vi "OpenLogFiles.vi"(8 "error in (no error)":errorcluster, 11 "WORef":T1) -> (0 "error out":errorcluster, 1 "FailRef":refnum<file>, 2 "PassRef":refnum<file>, 3 "WORef Out":T1)   [LabVIEW 2011]
uses:
  Classes/WorkorderHandler/Software/DataStructures/WorkorderHandler_ObjectReference.ctl
  Strict Type Controls/Settings Operation.ctl
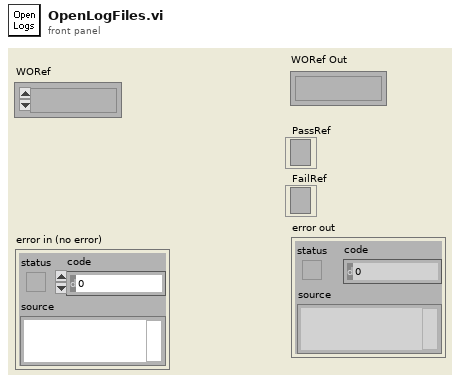
[diagram p1: front panel]
types:
  T1 = typedef "WorkorderHandler_ObjectReference.ctl" = refnum<k1>
  T2 = enum16{"open", "replace", "create", "open or create", "replace or create", "replace or create with confirmation"}
  T3 = typedef "Settings Operation.ctl" = enum8{"Get Value", "Set Value", "Read File", "Write File", "Write Stored Value"}
  T4 = cluster{"PassLog":path, "Fail Log":path, "Header":string, "LastSr":string}
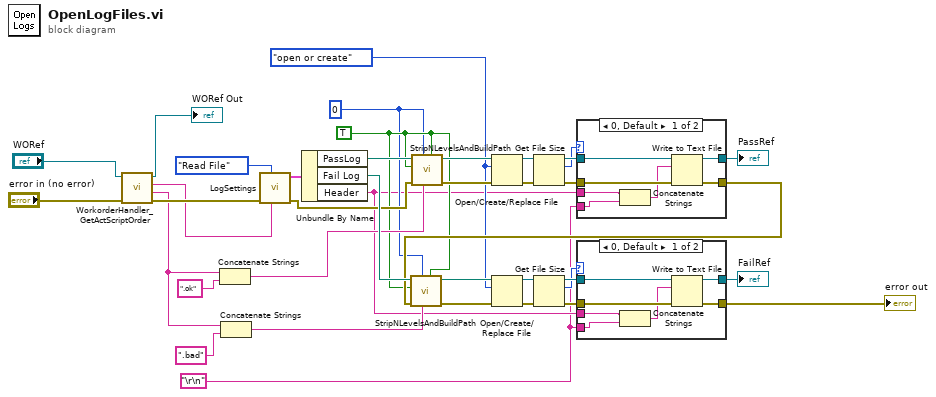
[diagram p0: block diagram]
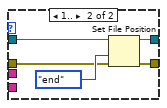
[diagram p2: hidden frame]
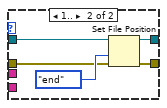
[diagram p3: hidden frame]
diagram:
  w9 = "\r\n"
  w14 = 0 ("Strip Levels")
  w15 = T2."open or create" ("operation (0:open)")
  w17 = TRUE ("Create Folders")
  n1 = call "WorkorderHandler_GetActScriptOrder.vi"("error in (no error)"="error in (no error)", "reference"="WORef") -> ("error out"=w4:errorcluster, "Order"=w2:string, "Script"=w3:string, "duplicate reference"=→"WORef Out":T1)  [unwired: 6 out]
  n2 = Concatenate Strings(w2, ".ok" ("string")) -> (w18:string)
  n3 = Concatenate Strings(w2, ".bad" ("string")) -> (w16:string)
  n4 = call "LogSettings.vi"("ScriptName"=w3, "Operation"=Settings_Operation."Read File", "error in (no error)"=w4) -> ("error out"=w22:errorcluster, "Settings out"=w37:T4)  [unwired: 1 in, 6 out]
  n5 = Unbundle By Name(w37) -> ("PassLog"=w31:path, "Fail Log"=w29:path, "Header"=w10:string)
  n6 = call "StripNLevelsAndBuildPath.vi"("Create Folders"=w17, "Build Path"=w18, "Strip Levels"=w14, "error in(no error)"=w22, "Is File"=w17, "Path In"=w31) -> ("error out"=w27:errorcluster, "Path Out"=w30:path)  [unwired: 4 out]
  n7 = Open/Create/Replace File(file path (use dialog)=w30, error in=w27, operation (0:open)=w15) -> (refnum out=w36:refnum<file>, error out=w26:errorcluster)  [unwired: 4 out]
  n8 = Get File Size(file=w36, error in=w26) -> (refnum out=w35:refnum<file>, size (in bytes)=w34:i64, 0:w23:errorcluster)
  n9 = case shown="0, Default" w34 {
    tunnel: w35 -> [w45 w50]
    tunnel: [w44 w48] -> w33
    tunnel: w10 -> [w40 _]
    tunnel: w23 -> [w43 w47]
    tunnel: [w42 w46] -> w21
    tunnel: w9 -> [w41 _]
    frame 0, Default {
      n10 = Concatenate Strings(w40, w41) -> (w39:string)
      n11 = Write to Text File(file (use dialog)=w45, text=w39, error in=w43) -> (refnum out=w44:refnum<file>, error out=w42:errorcluster)  [unwired: 2 out]
    }
    frame 1.. {
      n12 = Set File Position(refnum=w50, from (0:start)=enum16{"start", "end", "current"}."end", error in=w47) -> (refnum out=w48:refnum<file>, error out=w46:errorcluster)  [unwired: 1 out]
    }
  }
  "PassRef" <- w33
  n13 = call "StripNLevelsAndBuildPath.vi"("Create Folders"=w17, "Build Path"=w16, "Strip Levels"=w14, "error in(no error)"=w21, "Is File"=w17, "Path In"=w29) -> ("error out"=w25:errorcluster, "Path Out"=w28:path)  [unwired: 4 out]
  n14 = Open/Create/Replace File(file path (use dialog)=w28, error in=w25, operation (0:open)=w15) -> (refnum out=w32:refnum<file>, error out=w24:errorcluster)  [unwired: 4 out]
  n15 = Get File Size(file=w32, error in=w24) -> (refnum out=w13:refnum<file>, size (in bytes)=w12:i64, 0:w11:errorcluster)
  n16 = case shown="0, Default" w12 {
    tunnel: w13 -> [w57 w62]
    tunnel: [w56 w60] -> w7
    tunnel: w10 -> [w52 _]
    tunnel: w11 -> [w55 w59]
    tunnel: [w54 w58] -> w8
    tunnel: w9 -> [w53 _]
    frame 0, Default {
      n17 = Concatenate Strings(w52, w53) -> (w51:string)
      n18 = Write to Text File(file (use dialog)=w57, text=w51, error in=w55) -> (refnum out=w56:refnum<file>, error out=w54:errorcluster)  [unwired: 2 out]
    }
    frame 1.. {
      n19 = Set File Position(refnum=w62, from (0:start)=enum16{"start", "end", "current"}."end", error in=w59) -> (refnum out=w60:refnum<file>, error out=w58:errorcluster)  [unwired: 1 out]
    }
  }
  "FailRef" <- w7
  "error out" <- w8
